vi "MoveDst.vi"(11 "DesiredDistance":dbl) -> ()   [LabVIEW 2016]
uses:
  <vilib>/addons/control/pid/NI_PID_pid.lvlib
panel:
  out "setpoint":dbl format="%.2f"
  in  "setpoint profile":cluster{"time (s)":dbl, "setpoint":dbl}[](array[cluster]) {"setpoint" format="%.2f"; "time (s)" format="%.3f"}
  in  "Wheel Diameter (m)":dbl
  in  "Coeff Frict":dbl
  in  "Robot Weight (kg)":dbl
  # "Robot weight is 150 lbs"
  # "Wheel Diam 4in"
  # "Coeff friction of floor is 1.3"
  # "68.03 kg"
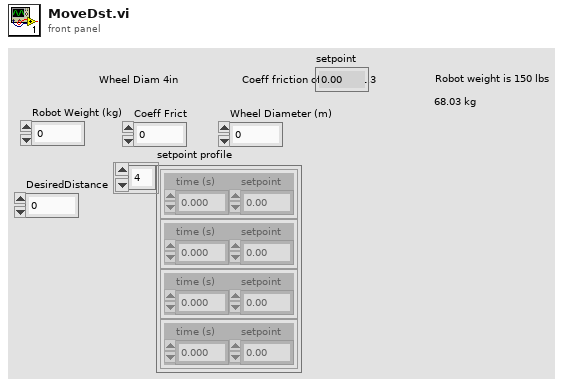
[diagram p1: front panel]
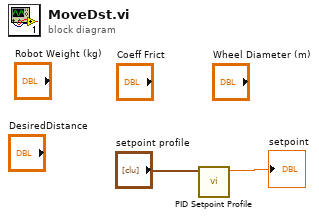
[diagram p0: block diagram]
diagram:
  n1 = call <vilib>:"PID Setpoint Profile.vi"("setpoint profile"="setpoint profile") -> ("setpoint"=→"setpoint":dbl)  [unwired: 5 in, 3 out]
